vi "Simple DAQ.vi"() -> ()   [LabVIEW 2015]
uses:
  Classes/DAQ/DAQ Parameters.ctl
  Classes/DAQ/Trigger Source.ctl
  Classes/DAQ/Trigger Slope.ctl
  Type Defs/OCT DAQ Channel Data Type.ctl
  Classes/DAQ/Clock Control.ctl
  Simple DAQ State.ctl
  ATS-VI/ATS_ctl/ATS_Check_Ctrl.ctl
  ATS-VI/ATS_ctl/Device_Ctrl.ctl
  Classes/DAQ/ATS660/ATS660 Class.lvclass
  Classes/DAQ/ATS9462/ATS9462 Class.lvclass
  Classes/DAQ/ATS9350/ATS9350.lvclass
  Classes/Laser/Insite/Insight.lvclass
  Classes/DAQ/DAQ Control Functional Global States.ctl
  <vilib>/Analysis/4window.llb/Hanning Window (DBL).vi
  <vilib>/Analysis/2dsp.llb/Real FFT.vi
  <vilib>/Analysis/4window.llb/AllCosWindow (DBL).vi
  Classes/DAQ/DAQ Class.lvclass
  <vilib>/Analysis/NI_AALPro.lvlib
panel:
  out "Path append":string="\\Insight LASER\\"
  in  "Record Data":bool
  in  "LASER Source":enum16{"INSIGHT", "SANTEC"}(ring)
  out "offset":dbl format="%.2f"
  out "mult":dbl
  in  "FFT Display":bool
  out "Frequency Domain":dbl[][](graph)
  in  "Pause Button":bool
  in  "Stop Button":bool
  in  "Play Button":bool
  out "Time Domain":dbl[][](graph)
  in  "DAQ Parameters Out":T1={"Points Per A-Scan"=1024, "A-Scans Per B-Scan"=250, "Number of B-Scans"=1, "A-Scans Per Transfer"=250, "Trigger Voltage"=200.0, "Trigger Source"=enum."External", "Trigger Slope"=enum."Rising", "Channel"=enum."Channel 1", "Clock"=enum."External Clock", "Bits per Sample"=16.0, "Range"=2.0}
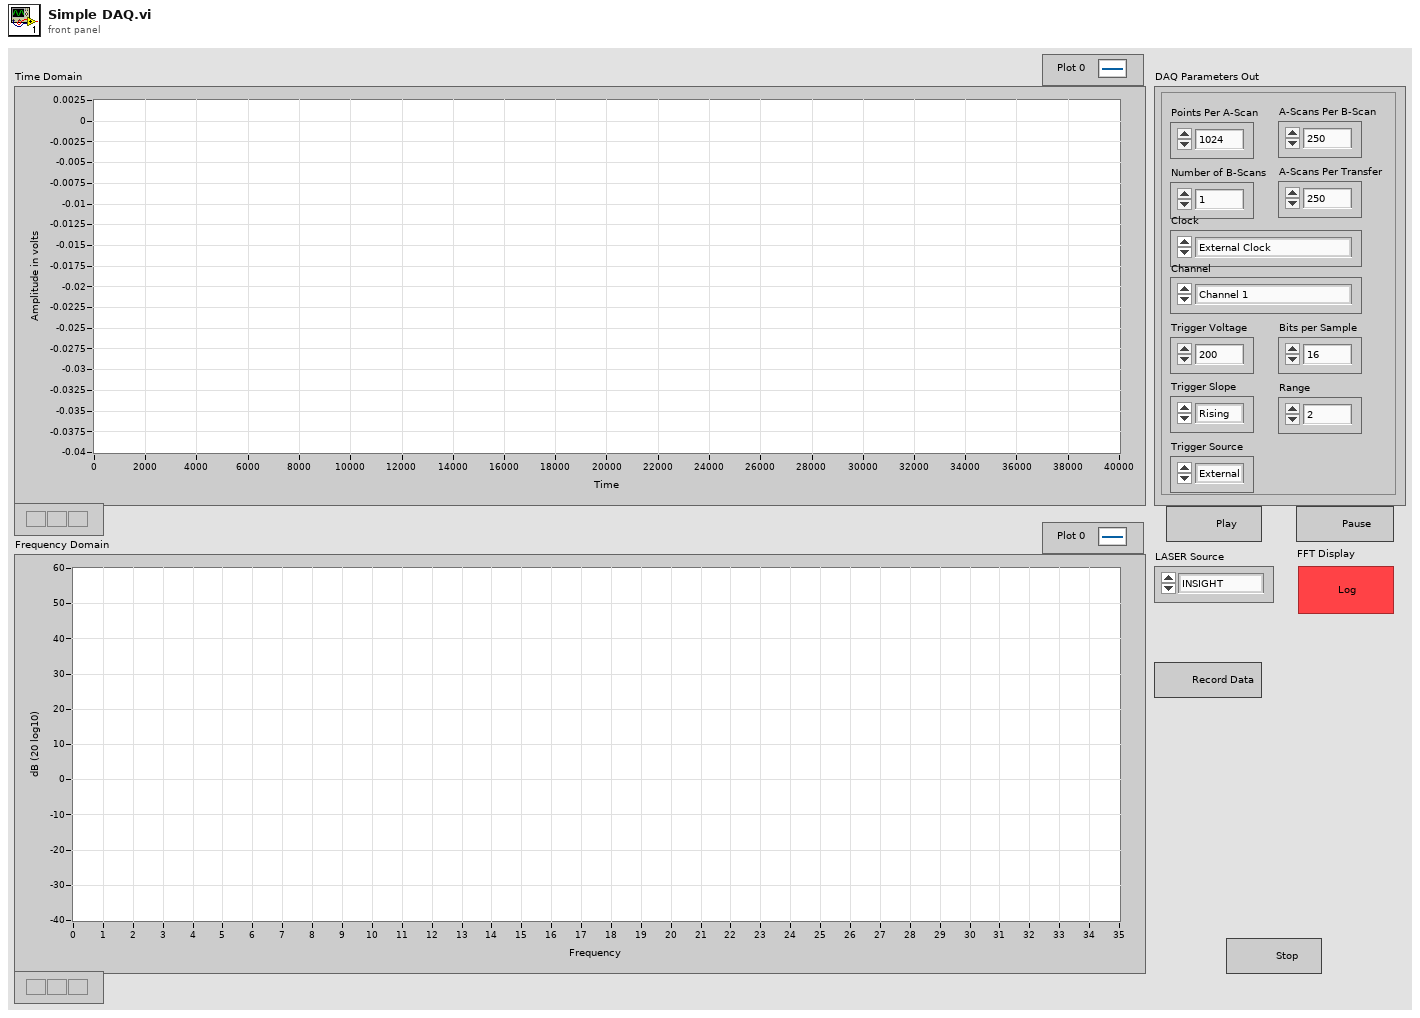
[diagram p1: front panel]
types:
  T1 = typedef "DAQ Class.lvclass/DAQ Parameters.ctl" = cluster{"Points Per A-Scan":u32, "A-Scans Per B-Scan":u32, "Number of B-Scans":u32, "A-Scans Per Transfer":u32, "Trigger Voltage":sgl, "Trigger Source":T2, "Trigger Slope":T3, "Channel":T4, "Clock":T5, "Bits per Sample":dbl, "Range":dbl}
  T2 = typedef "DAQ Class.lvclass/Trigger Source.ctl" = enum16{"External", "Channel A", "Channel B"}
  T3 = typedef "DAQ Class.lvclass/Trigger Slope.ctl" = enum16{"Rising", "Falling"}
  T4 = typedef "OCT DAQ Channel Data Type.ctl" = enum16{"Channel 1", "Channel 2", "Channel 1 and 2"}
  T5 = typedef "DAQ Class.lvclass/Clock Control.ctl" = enum16{"Internal Clock", "External Clock"}
  T6 = typedef "Device_Ctrl.ctl" = enum16{"Status", "About", "Arm", "ForceTrig", "Abort", "Initialize", "Init (NoPreset)", "Info", "Close", "Calibrate", "SetManually", "LED_ON", "LED_OFF"}
  T7 = typedef "ATS_Check_Ctrl.ctl" = enum16{"None", "NO_ATS9462", "ATS9462_Traditional", "Verify Board", "OnBoard Memory", "Board & Memory", "Master/Slave", "NO Master/Slave"}
  T8 = typedef "Simple DAQ State.ctl" = enum16{"Initialize DAQ", "Reset DAQ", "Configure DAQ", "Acquire", "Acquire and Save", "Stop"}
  T9 = typedef "Device_Info.ctl" = cluster{"Handle":u32, "Board":string, "CPLD":string, "MemorySize":u32, "SampleSize":u8, "ID":i32, "High_Memory":bool, "Chan/Board":u8}
  T10 = typedef "DAQ Control Functional Global States.ctl" = enum16{"Status", "Set Processing Finished", "Reset", "Clear", "Set DAQ Finished"}
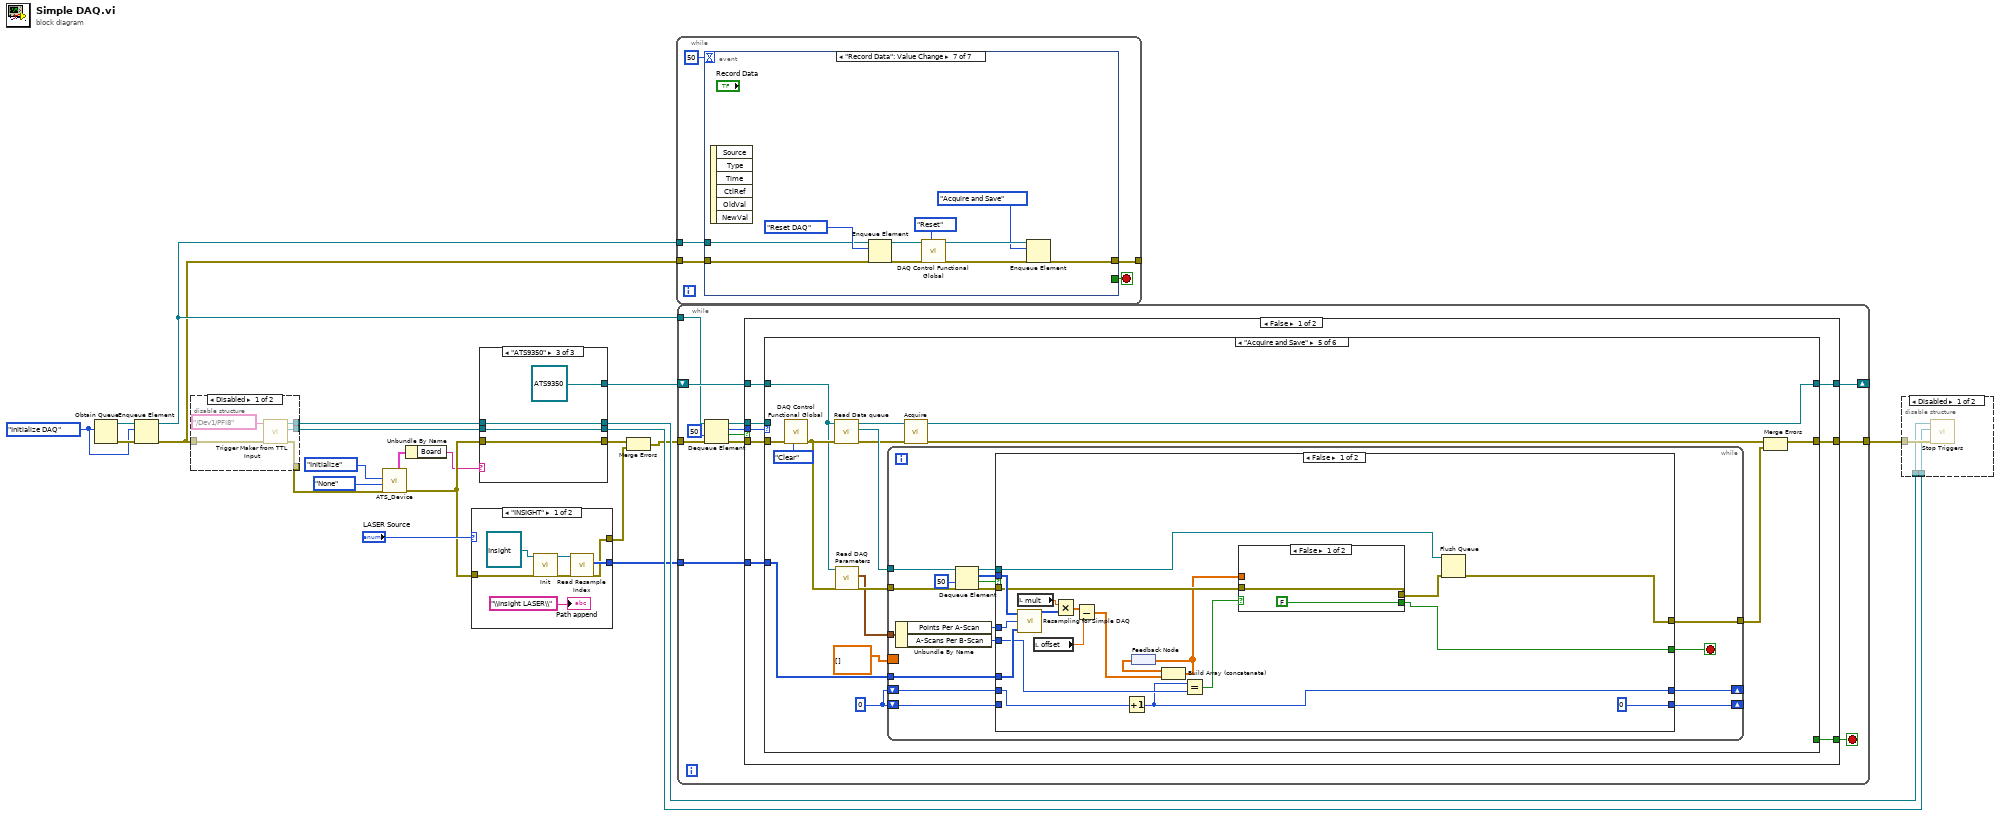
[diagram p0: block diagram]
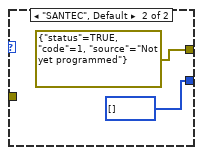
[diagram p4: hidden frame]
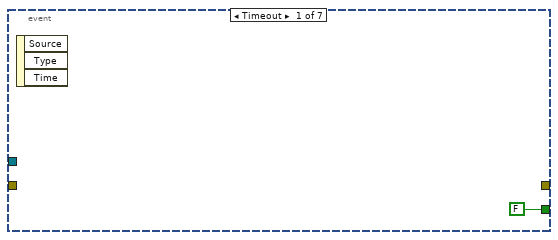
[diagram p5: hidden frame]
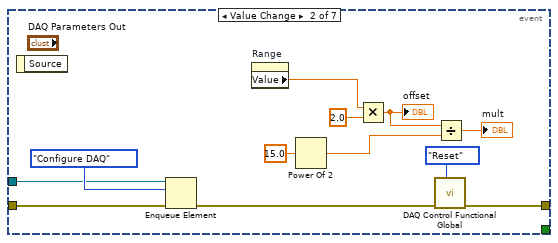
[diagram p6: hidden frame]
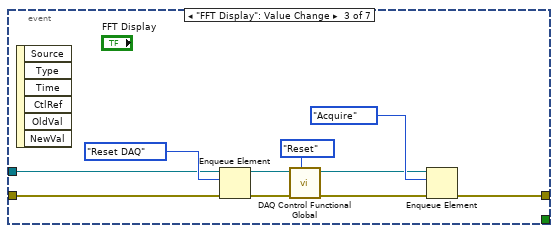
[diagram p7: hidden frame]
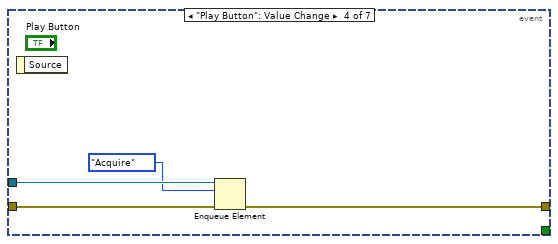
[diagram p8: hidden frame]
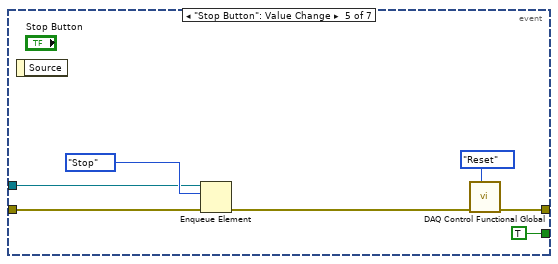
[diagram p9: hidden frame]
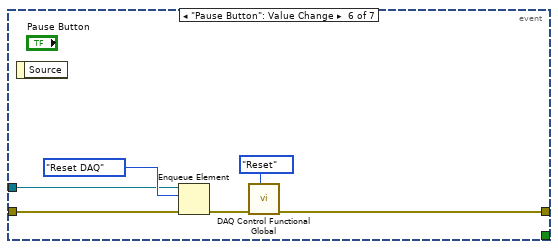
[diagram p10: hidden frame]
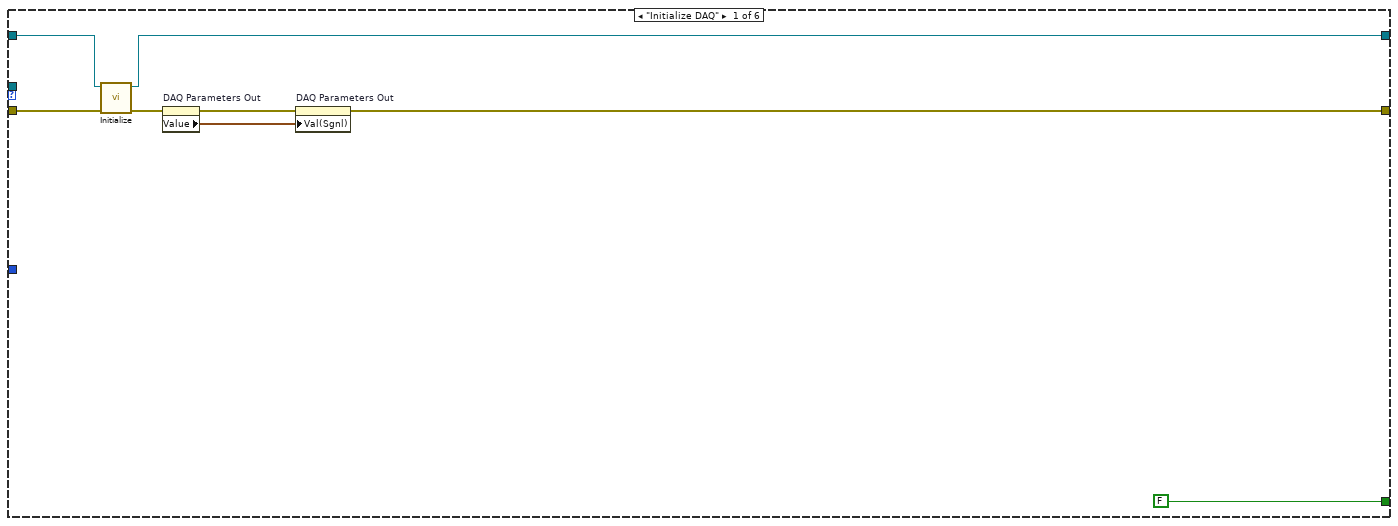
[diagram p11: hidden frame]
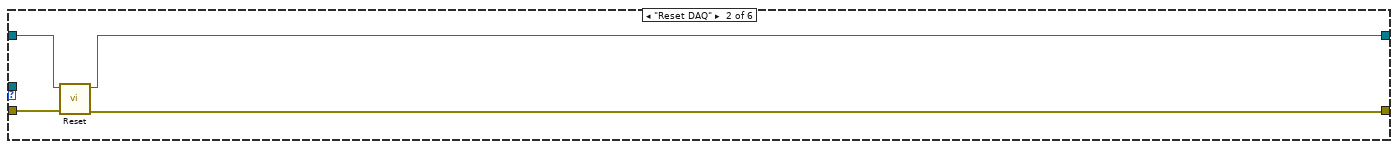
[diagram p12: hidden frame]
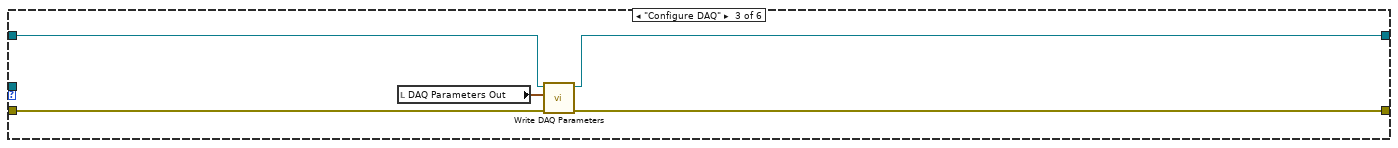
[diagram p13: hidden frame]
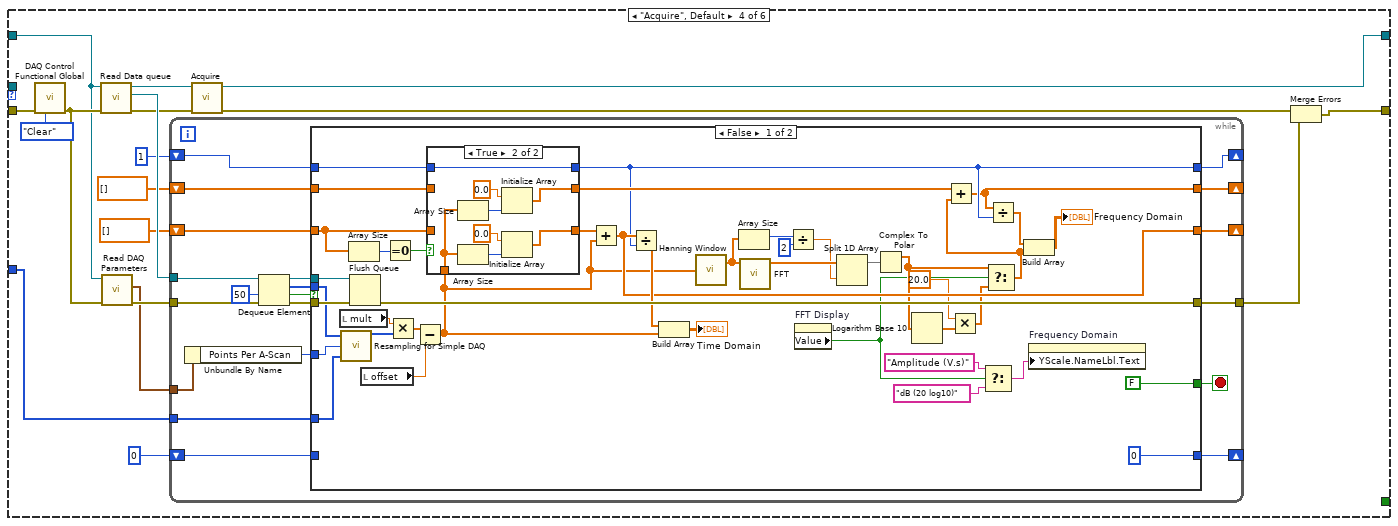
[diagram p14: hidden frame]
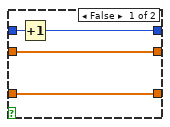
[diagram p15: hidden frame]
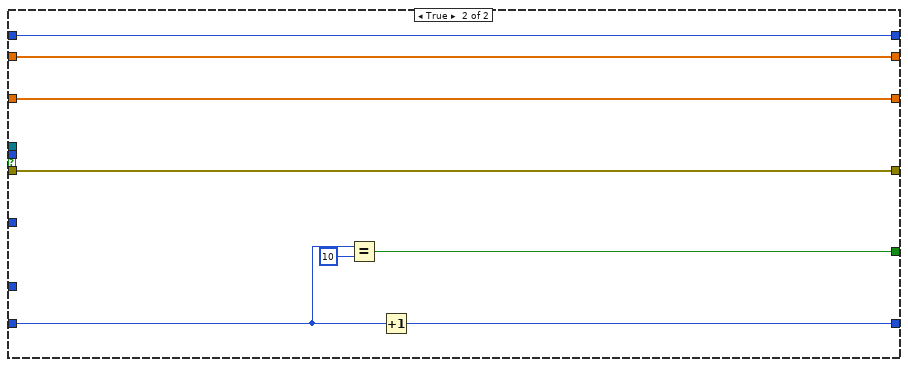
[diagram p16: hidden frame]
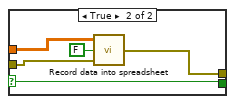
[diagram p17: hidden frame]
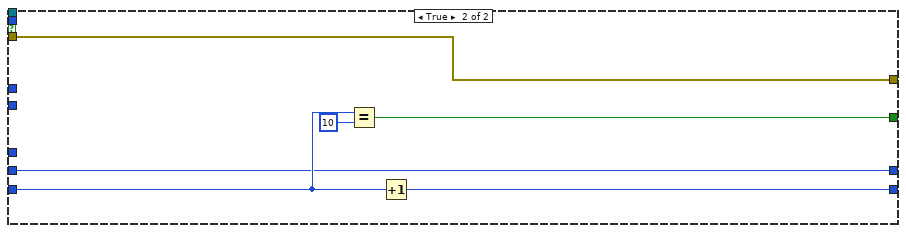
[diagram p18: hidden frame]
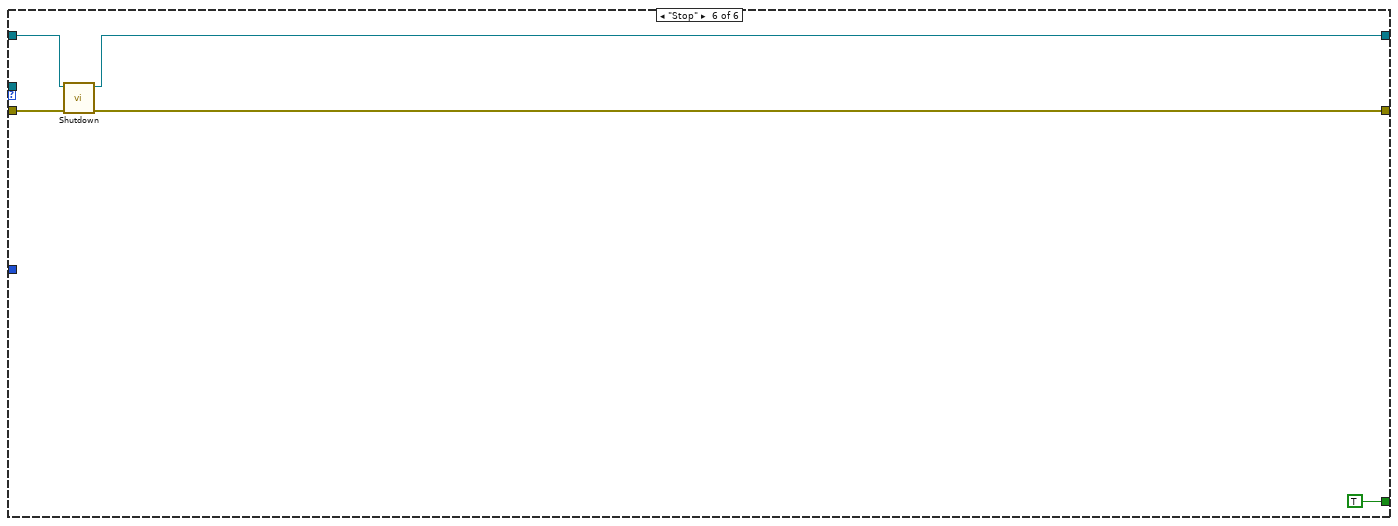
[diagram p19: hidden frame]
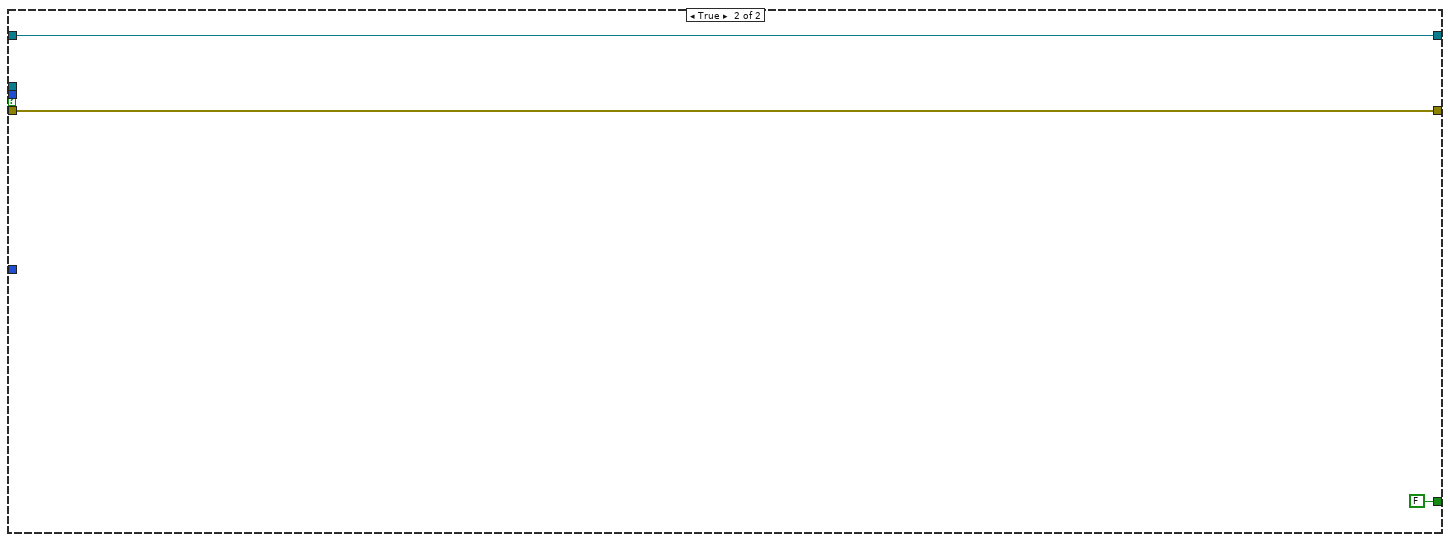
[diagram p20: hidden frame]
diagram:
  w11 = Simple_DAQ_State."Initialize DAQ" ("Simple OCT States")
  n1 = Obtain Queue(element data type=w11) -> (queue out=w15:refnum<queue>, error out=w14:errorcluster)  [unwired: 4 in, 1 out]
  n2 = Enqueue Element(queue=w15, element=w11, error in (no error)=w14) -> (queue out=w13:refnum<queue>, error out=w12:errorcluster)  [unwired: 1 in, 1 out]
  n3 = disable-structure shown="Disabled" {
    disable-tunnel: [w26 _] -> w22
    disable-tunnel: [w25 _] -> w21
    disable-tunnel: w12 -> [w24 _]
    disable-tunnel: [w23 _] -> w3
    frame Disabled {
      n4 = call "Trigger Maker from TTL Input.vi"("Error in"=w24, "Master Trigger In from Laser (TTL)"=tag "/Dev1/PFI8") -> ("error out"=w23:errorcluster, "Alazar Task"=w25:refnum<k21>, "AFG11000 Task"=w26:refnum<k21>)  [unwired: 7 in]
    }
    frame Enabled {
    }
  }
  n5 = call "ATS_Device.vi"("error in (no error)"=w3, "ATS_Check"=ATS_Check_Ctrl."None", "DevCtrl"=Device_Ctrl."Initialize") -> ("error out"=w2:errorcluster, "DevInfo"=w6:T9)  [unwired: 2 in, 5 out]
  n6 = Unbundle By Name(w6) -> ("Board"=w1:string)
  n7 = case shown="\"INSIGHT\"" "LASER Source" {
    tunnel: w2 -> [w28 _]
    tunnel: [w34 u32[] [] ("Resample Index")] -> w9
    tunnel: [w33 errorcluster {"status"=TRUE, "code"=1, "source"="Not yet programmed"} ("error constant")] -> w7
    frame "INSIGHT" {
      n8 = call-dynamic "Init.vi"("error in (no error)"=w28, "Insite in"=refnum<class "Insight.lvclass"> refnum ("Insight.lvclass")) -> ("error out"=w29:errorcluster, "Insite out"=w30:refnum<class "Insight.lvclass">)  [unwired: 8 in]
      n9 = call-dynamic "Read Resample Index.vi"("error in (no error)"=w29, "Laser in"=w30) -> ("error out"=w33:errorcluster, "Resample Index"=w34:u32[])  [unwired: 7 in, 1 out]
      "Path append" <- "\\Insight LASER\\"
    }
    frame "SANTEC", Default {
    }
  }
  n10 = case shown="\"ATS9350\"" w1 {
    tunnel: w2 -> [w38 w41 w46]
    tunnel: [w40 w43 w48] -> w17
    tunnel: w22 -> [w40 w43 w48]
    tunnel: w21 -> [w39 w42 w47]
    tunnel: [w39 w42 w47] -> w16
    tunnel: [w38 w41 w46] -> w20
    tunnel: [refnum<class "ATS660 Class.lvclass"> refnum ("ATS660 Class.lvclass") refnum<class "ATS9462 Class.lvclass"> refnum ("ATS9462 Class.lvclass") refnum<class "ATS9350.lvclass"> refnum ("ATS9350.lvclass")] -> w19
    frame "ATS660", Default {
    }
    frame "ATS9462" {
    }
    frame "ATS9350" {
    }
  }
  n11 = Merge Errors(w20, w7) -> (w8:errorcluster)
  n12 = while {
    tunnel: w13 -> [w50]
    tunnel: w12 -> [w51]
    tunnel: [w49] -> _
    stop <- w53 stop-if-true
    n13 = event shown="[6] \"Record Data\": Value Change" {
      selector: _ -> [_ _ _ _ _ _ _]
      dyn-events: _ -> [_ _ _ _ _ _ _]
      timeout: 50 -> [_ _ _ _ _ _ _]
      tunnel: [FALSE _ _ _ TRUE _ _] -> w53
      tunnel: w51 -> [_ w63 w71 w78 w81 w91 w94]
      tunnel: w50 -> [_ w64 w72 w79 w80 w90 w95]
      tunnel: [_ w61 w69 w77 w82 w87 w93] -> w49
      event Timeout {
        n14 = event-data() -> ()  [unwired: 1 in, 3 out]
      }
      event Value Change {
        n15 = event-data() -> ()  [unwired: 1 in, 1 out]
        n16 = Enqueue Element(queue=w64, element=Simple_DAQ_State."Configure DAQ" ("Simple OCT States"), error in (no error)=w63) -> (error out=w62:errorcluster)  [unwired: 1 in, 2 out]
        n17 = property on="Range" class="DigNum (strict)"() -> ("Value"=w56:dbl)  [unwired: 2 in, 2 out]
        n18 = Power Of 2(x=15.0) -> (2^x=w59:dbl)
        n19 = Multiply(x=w56, y=2.0 ("Offset")) -> (x*y=w55:dbl)
        "offset" <- w55
        n20 = call "DAQ Control Functional Global.vi"("State"=DAQ_Control_Functional_Global_States."Reset", "Error In"=w62) -> ("Error Out"=w61:errorcluster)  [unwired: 6 in, 3 out]
        n21 = Divide(x=w55, y=w59) -> (x/y=→"mult":dbl)
      }
      event "FFT Display": Value Change {
        n22 = event-data() -> ()  [unwired: 1 in, 6 out]
        n23 = Enqueue Element(queue=w72, element=Simple_DAQ_State."Reset DAQ" ("Simple OCT States"), error in (no error)=w71) -> (queue out=w67:refnum<queue>, error out=w75:errorcluster)  [unwired: 1 in, 1 out]
        n24 = call "DAQ Control Functional Global.vi"("State"=DAQ_Control_Functional_Global_States."Reset", "Error In"=w75) -> ("Error Out"=w68:errorcluster)  [unwired: 6 in, 3 out]
        n25 = Enqueue Element(queue=w67, element=Simple_DAQ_State."Acquire" ("Simple OCT States"), error in (no error)=w68) -> (error out=w69:errorcluster)  [unwired: 1 in, 2 out]
      }
      event "Play Button": Value Change {
        n26 = event-data() -> ()  [unwired: 1 in, 1 out]
        n27 = Enqueue Element(queue=w79, element=Simple_DAQ_State."Acquire" ("Simple OCT States"), error in (no error)=w78) -> (error out=w77:errorcluster)  [unwired: 1 in, 2 out]
      }
      event "Stop Button": Value Change {
        n28 = event-data() -> ()  [unwired: 1 in, 1 out]
        n29 = Enqueue Element(queue=w80, element=Simple_DAQ_State."Stop" ("Simple OCT States"), error in (no error)=w81) -> (error out=w83:errorcluster)  [unwired: 1 in, 2 out]
        n30 = call "DAQ Control Functional Global.vi"("State"=DAQ_Control_Functional_Global_States."Reset", "Error In"=w83) -> ("Error Out"=w82:errorcluster)  [unwired: 6 in, 3 out]
      }
      event "Pause Button": Value Change {
        n31 = event-data() -> ()  [unwired: 1 in, 1 out]
        n32 = Enqueue Element(queue=w90, element=Simple_DAQ_State."Reset DAQ" ("Simple OCT States"), error in (no error)=w91) -> (error out=w88:errorcluster)  [unwired: 1 in, 2 out]
        n33 = call "DAQ Control Functional Global.vi"("State"=DAQ_Control_Functional_Global_States."Reset", "Error In"=w88) -> ("Error Out"=w87:errorcluster)  [unwired: 6 in, 3 out]
      }
      event "Record Data": Value Change {
        n34 = event-data() -> ()  [unwired: 1 in, 6 out]
        n35 = Enqueue Element(queue=w95, element=Simple_DAQ_State."Reset DAQ" ("Simple OCT States"), error in (no error)=w94) -> (queue out=w101:refnum<queue>, error out=w96:errorcluster)  [unwired: 1 in, 1 out]
        n36 = call "DAQ Control Functional Global.vi"("State"=DAQ_Control_Functional_Global_States."Reset", "Error In"=w96) -> ("Error Out"=w100:errorcluster)  [unwired: 6 in, 3 out]
        n37 = Enqueue Element(queue=w101, element=Simple_DAQ_State."Acquire and Save" ("Simple OCT States"), error in (no error)=w100) -> (error out=w93:errorcluster)  [unwired: 1 in, 2 out]
      }
    }
  }
  n38 = while {
    tunnel: w8 -> [w111]
    tunnel: w13 -> [w107]
    tunnel: [w104] -> w18
    shift-right: [w103] -> _
    shift-left: w19 -> [w113]
    tunnel: w9 -> [w102]
    stop <- w112 stop-if-true
    n39 = Dequeue Element(queue=w107, timeout in ms (-1)=50, error in (no error)=w111) -> (queue out=w106:refnum<queue>, element=w105:T8, timed out?=w108:bool, error out=w110:errorcluster)
    n40 = case shown="False" w108 {
      tunnel: w110 -> [w121 w312]
      tunnel: w113 -> [w120 w310]
      tunnel: [w118 FALSE] -> w112
      tunnel: w106 -> [w115 _]
      tunnel: w105 -> [w119 _]
      tunnel: [w117 w312] -> w104
      tunnel: [w116 w310] -> w103
      tunnel: w102 -> [w114 _]
      frame False {
        n41 = case shown="\"Acquire and Save\"" w119 {
          tunnel: w121 -> [w129 w133 w138 w148 w249 w309]
          tunnel: w120 -> [w128 w132 w137 w142 w244 w308]
          tunnel: [FALSE _ _ _ _ TRUE] -> w118
          tunnel: [w122 w130 w135 w146 w247 w306] -> w117
          tunnel: [w126 w131 w134 w147 w248 w307] -> w116
          tunnel: w115 -> [_ _ _ _ _ _]
          tunnel: w114 -> [_ _ _ w139 w242 _]
          frame "Initialize DAQ" {
            n42 = call-dynamic "Initialize.vi"("error in (no error)"=w129, "DAQ Class in"=w128) -> ("error out"=w125:errorcluster, "DAQ Class out"=w126:refnum<class "DAQ Class.lvclass">)  [unwired: 8 in]
            n43 = property on="DAQ Parameters Out" class="Clust (strict)"(error in=w125) -> (error out=w124:errorcluster, "Value"=w123:T1)  [unwired: 1 in, 1 out]
            n44 = property on="DAQ Parameters Out" class="Clust (strict)"(error in=w124, "Val(Sgnl)"=w123) -> (error out=w122:errorcluster)  [unwired: 1 in, 1 out]
          }
          frame "Reset DAQ" {
            n45 = call-dynamic "Reset.vi"("error in (no error)"=w133, "DAQ Class in"=w132) -> ("error out"=w130:errorcluster, "DAQ Class out"=w131:refnum<class "DAQ Class.lvclass">)  [unwired: 8 in]
          }
          frame "Configure DAQ" {
            n46 = local read "DAQ Parameters Out"() -> (w136:T1)
            n47 = call-dynamic "Write DAQ Parameters.vi"("error in (no error)"=w138, "DAQ Parameters"=w136, "DAQ Class in"=w137) -> ("error out"=w135:errorcluster, "DAQ Class out"=w134:refnum<class "DAQ Class.lvclass">)  [unwired: 7 in]
          }
          frame "Acquire", Default {
            n48 = call "DAQ Control Functional Global.vi"("State"=DAQ_Control_Functional_Global_States."Clear", "Error In"=w148) -> ("Error Out"=w143:errorcluster)  [unwired: 6 in, 3 out]
            n49 = call-dynamic "Read Data queue.vi"("error in (no error)"=w143, "DAQ Class in"=w142) -> ("error out"=w154:errorcluster, "Data queue"=w155:refnum<queue>, "DAQ Class out"=w156:refnum<class "DAQ Class.lvclass">)  [unwired: 7 in]
            n50 = call-dynamic "Read DAQ Parameters.vi"("error in (no error)"=w143, "DAQ Class in"=w142) -> ("error out"=w144:errorcluster, "DAQ Parameters"=w141:T1)  [unwired: 7 in, 1 out]
            n51 = while {
              tunnel: w155 -> [w176]
              tunnel: w144 -> [w175]
              shift-right: [w167] -> _
              shift-left: sgl[] [] -> [w172]
              shift-right: [w165] -> _
              shift-left: 1 -> [w166]
              tunnel: [w164] -> w151
              shift-right: [w162] -> _
              shift-left: 0 -> [w163]
              tunnel: w141 -> [w161]
              shift-right: [w159] -> _
              shift-left: sgl[] [] -> [w160]
              tunnel: w139 -> [w158]
              stop <- w173 stop-if-true
              n52 = Unbundle By Name(w161) -> ("Points Per A-Scan"=w157:u32)
              n53 = Dequeue Element(queue=w176, timeout in ms (-1)=50, error in (no error)=w175) -> (queue out=w169:refnum<queue>, element=w168:u16[], timed out?=w171:bool, error out=w170:errorcluster)
              n54 = case shown="False" w171 {
                tunnel: [FALSE w232] -> w173
                tunnel: w172 -> [w214 w238]
                tunnel: w170 -> [w217 w236]
                tunnel: w169 -> [w218 _]
                tunnel: w168 -> [w208 _]
                tunnel: [w204 w238] -> w167
                tunnel: w166 -> [w212 w237]
                tunnel: [w195 w237] -> w165
                tunnel: [w211 w236] -> w164
                tunnel: w163 -> [_ w234]
                tunnel: [0 w235] -> w162
                tunnel: w157 -> [w207 _]
                tunnel: w160 -> [w203 w231]
                tunnel: [w194 w231] -> w159
                tunnel: w158 -> [w177 _]
                frame False {
                  n55 = local read "mult"() -> (w180:dbl)
                  n56 = call "Resampling for Simple DAQ.vi"("Resample Index"=w177, "Points Per A-Scan"=w207, "U16 Array"=w208) -> ("Array"=w181:u16[])
                  n57 = Array Size(array=w214) -> (size(s)=w216:i32)
                  n58 = Flush Queue(queue=w218, error in (no error)=w217) -> (error out=w211:errorcluster)  [unwired: 2 out]
                  n59 = local read "offset"() -> (w179:dbl)
                  n60 = Equal To 0?(x=w216) -> (x = 0?=w215:bool)
                  n61 = Multiply(x=w180, y=w181) -> (x*y=w182:dbl[])
                  n62 = Subtract(x=w182, y=w179) -> (x-y=w178:dbl[])
                  n63 = case shown="True" w215 {
                    tunnel: w178 -> [_ w223]
                    tunnel: w214 -> [w222 _]
                    tunnel: [w222 w228] -> w213
                    tunnel: w212 -> [w221 w227]
                    tunnel: [w220 w227] -> w195
                    tunnel: w203 -> [w219 _]
                    tunnel: [w219 w224] -> w199
                    frame False {
                      n64 = Increment(x=w221) -> (x+1=w220:i32)
                    }
                    frame True {
                      n65 = Array Size(array=w223) -> (size(s)=w225:i32)
                      n66 = Array Size(array=w223) -> (size(s)=w230:i32)
                      n67 = Initialize Array(sgl 0.0 ("element"), w225) -> (w224:sgl[])
                      n68 = Initialize Array(sgl 0.0 ("element"), w230) -> (w228:sgl[])
                    }
                  }
                  n69 = Add(x=w213, y=w178) -> (x+y=w204:dbl[])
                  n70 = Divide(x=w204, y=w195) -> (x/y=w206:dbl[])
                  n71 = Build Array(w206, w178) -> (→"Time Domain":dbl[][])
                  n72 = call-poly <vilib>:"Hanning Window.vi"("X"=w178) -> ("Windowed X"=w202:dbl[])  [unwired: 1 out]
                  n73 = Array Size(array=w202) -> (size(s)=w201:i32)
                  n74 = call-poly <vilib>:"FFT.vi"("X"=w202) -> ("FFT {X}"=w198:cdb[])  [unwired: 9 in, 1 out]
                  n75 = Divide(x=w201, y=2) -> (x/y=w197:dbl)
                  n76 = property on="FFT Display" class="Bool (strict)"() -> ("Value"=w183:bool)  [unwired: 2 in, 2 out]
                  n77 = Split 1D Array(array=w198, index=w197) -> (first subarray=w196:cdb[])  [unwired: 1 out]
                  n78 = Complex To Polar(r * e^(i*theta)=w196) -> (r=w191:dbl[])  [unwired: 1 out]
                  n79 = Logarithm Base 10(1:w191) -> (0:w190:dbl[])
                  n80 = Multiply(x=20.0, y=w190) -> (x*y=w188:dbl[])
                  n81 = Select(t="Amplitude (V.s)", s=w183, f="dB (20 log10)") -> (s? t:f=w186:string)
                  n82 = Select(t=w191, s=w183, f=w188) -> (s? t:f=w187:dbl[])
                  n83 = Add(x=w199, y=w187) -> (x+y=w194:dbl[])
                  n84 = Divide(x=w194, y=w195) -> (x/y=w192:dbl[])
                  n85 = Build Array(w192, w187) -> (→"Frequency Domain":dbl[][])
                  n86 = property on="Frequency Domain" class="WFGraph (strict)"("YScale.NameLbl.Text"=w186) -> ()  [unwired: 2 in, 2 out]
                }
                frame True {
                  n87 = Equal?(x=w234, y=10) -> (x = y?=w232:bool)
                  n88 = Increment(x=w234) -> (x+1=w235:i32)
                }
              }
            }
            n89 = call-dynamic "Acquire.vi"("error in (no error)"=w154, "DAQ Class in"=w156) -> ("error out"=w150:errorcluster, "DAQ Class out"=w147:refnum<class "DAQ Class.lvclass">)  [unwired: 8 in]
            n90 = Merge Errors(w150, w151) -> (w146:errorcluster)
          }
          frame "Acquire and Save" {
            w241 = 0
            n91 = call "DAQ Control Functional Global.vi"("State"=DAQ_Control_Functional_Global_States."Clear", "Error In"=w249) -> ("Error Out"=w245:errorcluster)  [unwired: 6 in, 3 out]
            n92 = call-dynamic "Read Data queue.vi"("error in (no error)"=w245, "DAQ Class in"=w244) -> ("error out"=w252:errorcluster, "Data queue"=w253:refnum<queue>, "DAQ Class out"=w254:refnum<class "DAQ Class.lvclass">)  [unwired: 7 in]
            n93 = call-dynamic "Read DAQ Parameters.vi"("error in (no error)"=w245, "DAQ Class in"=w244) -> ("error out"=w246:errorcluster, "DAQ Parameters"=w243:T1)  [unwired: 7 in, 1 out]
            n94 = while {
              tunnel: w253 -> [w271]
              tunnel: w246 -> [w270]
              shift-right: [w263] -> _
              shift-left: w241 -> [w264]
              tunnel: w243 -> [w262]
              tunnel: w242 -> [w261]
              shift-right: [w257] -> _
              shift-left: w241 -> [w258]
              tunnel: [w255] -> w240
              border: dbl[][] [] -> [_]
              stop <- w256 stop-if-true
              n95 = Unbundle By Name(w262) -> ("Points Per A-Scan"=w260:u32, "A-Scans Per B-Scan"=w259:u32)
              n96 = Dequeue Element(queue=w271, timeout in ms (-1)=50, error in (no error)=w270) -> (queue out=w266:refnum<queue>, element=w265:u16[], timed out?=w268:bool, error out=w267:errorcluster)
              n97 = case shown="False" w268 {
                tunnel: [w274 w300] -> w256
                tunnel: w267 -> [w277 w304]
                tunnel: w266 -> [w291 _]
                tunnel: w265 -> [w290 _]
                tunnel: [w275 w304] -> w255
                tunnel: w264 -> [_ w302]
                tunnel: [0 w303] -> w263
                tunnel: w260 -> [w289 _]
                tunnel: w261 -> [w284 _]
                tunnel: w259 -> [w283 _]
                tunnel: w258 -> [w281 w299]
                tunnel: [w280 w299] -> w257
                frame False {
                  n98 = local read "mult"() -> (w286:dbl)
                  n99 = call "Resampling for Simple DAQ.vi"("Resample Index"=w284, "Points Per A-Scan"=w289, "U16 Array"=w290) -> ("Array"=w287:u16[])
                  n100 = local read "offset"() -> (w285:dbl)
                  n101 = Multiply(x=w286, y=w287) -> (x*y=w288:dbl[])
                  n102 = Subtract(x=w288, y=w285) -> (x-y=w279:dbl[])
                  n103 = Increment(x=w281) -> (x+1=w280:i32)
                  n104 = feedback #1() -> (w272:dbl[][])
                  n105 = Build Array (concatenate)(w272, w279) -> (w273:dbl[][])
                  n106 = feedback-in #1(w273) -> ()
                  n107 = Equal?(x=w280, y=w283) -> (x = y?=w278:bool)
                  n108 = case shown="False" w278 {
                    selector: w278 -> [_ w294]
                    tunnel: w277 -> [w293 w296]
                    tunnel: [w293 w298] -> w276
                    tunnel: w273 -> [_ w297]
                    tunnel: [FALSE w294] -> w274
                    frame False {
                    }
                    frame True {
                      n109 = call "Record data into spreadsheet.vi"("Error In"=w296, "Append?"=FALSE, "Data"=w297) -> ("Error Out"=w298:errorcluster)
                    }
                  }
                  n110 = Flush Queue(queue=w291, error in (no error)=w276) -> (error out=w275:errorcluster)  [unwired: 2 out]
                }
                frame True {
                  n111 = Equal?(x=w302, y=10) -> (x = y?=w300:bool)
                  n112 = Increment(x=w302) -> (x+1=w303:i32)
                }
              }
            }
            n113 = call-dynamic "Acquire.vi"("error in (no error)"=w252, "DAQ Class in"=w254) -> ("error out"=w251:errorcluster, "DAQ Class out"=w248:refnum<class "DAQ Class.lvclass">)  [unwired: 8 in]
            n114 = Merge Errors(w251, w240) -> (w247:errorcluster)
          }
          frame "Stop" {
            n115 = call-dynamic "Shutdown.vi"("error in (no error)"=w309, "DAQ Class in"=w308) -> ("error out"=w306:errorcluster, "DAQ Class out"=w307:refnum<class "DAQ Class.lvclass">)  [unwired: 8 in]
          }
        }
      }
      frame True {
      }
    }
  }
  n116 = disable-structure shown="Disabled" {
    disable-tunnel: w18 -> [w315 _]
    disable-tunnel: w17 -> [w314 _]
    disable-tunnel: w16 -> [w313 _]
    frame Disabled {
      n117 = call "Stop Triggers.vi"("Error in"=w315, "Alazar Task"=w313, "AFG11000 Task"=w314) -> ()  [unwired: 8 in, 1 out]
    }
    frame Enabled {
    }
  }
